vi "TIMER_VI.vi"(7 "simulazione":bool, 8 "error in (no error)":errorcluster, 11 "Queue Name":string) -> (0 "error out":errorcluster, 2 "Stopped":bool)   [LabVIEW 2019]
uses:
  Globals.vi
panel:
  out "# elements in queue":i32
  out "Elapsed Time (s)":dbl
  out "STATO":string
  out "LOOP TIME (ms)":u32
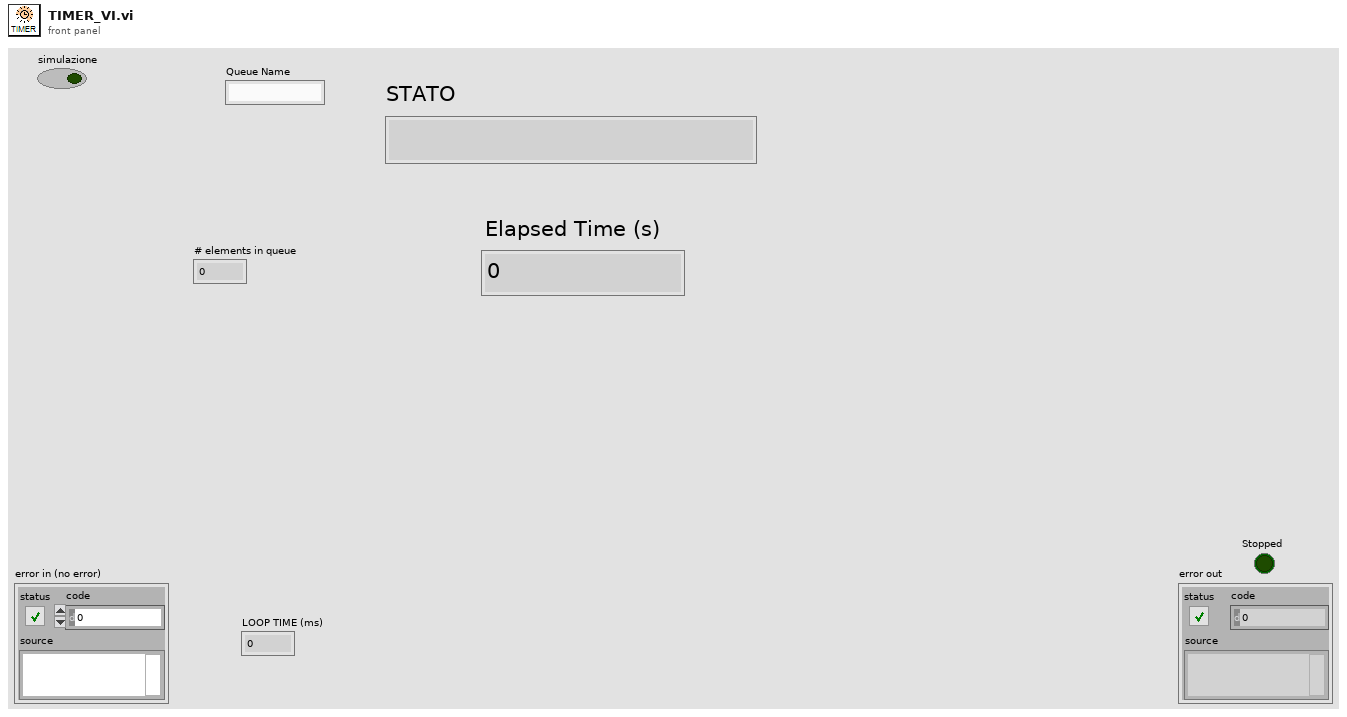
[diagram p1: front panel]
types:
  T1 = cluster{"Array of elements":cluster{"String":string, "variant":variant}[], "Single element":cluster{"String":string, "variant":variant}, "enque at\nopposite end (F)":bool, "no replications (F)":bool}
  T2 = enum32{"Invalid", "Standard", "Closed", "Hidden", "Minimized", "Maximized"}
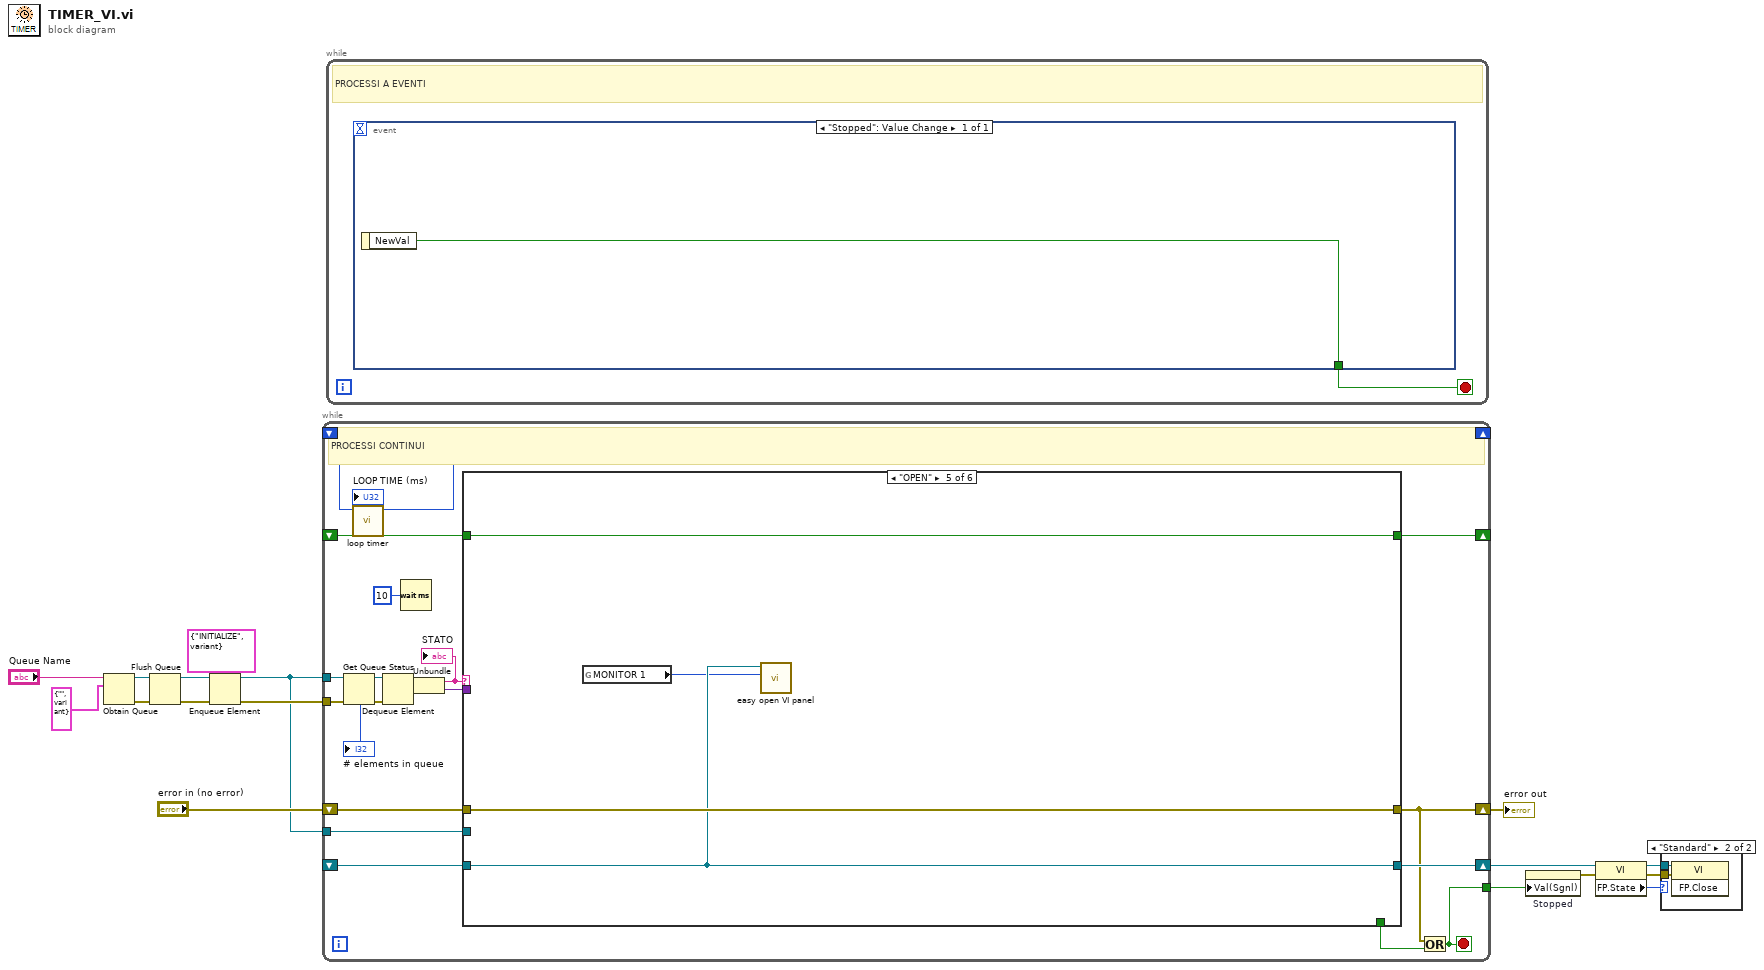
[diagram p0: block diagram]
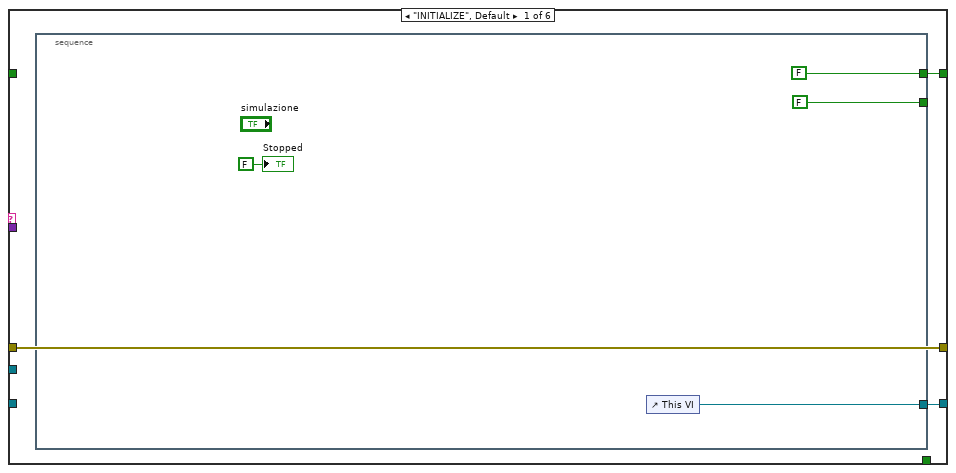
[diagram p3: hidden frame]
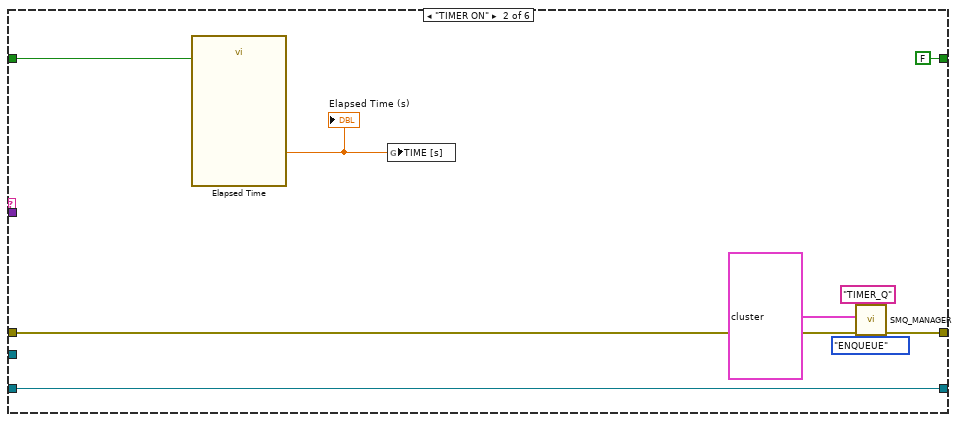
[diagram p4: hidden frame]
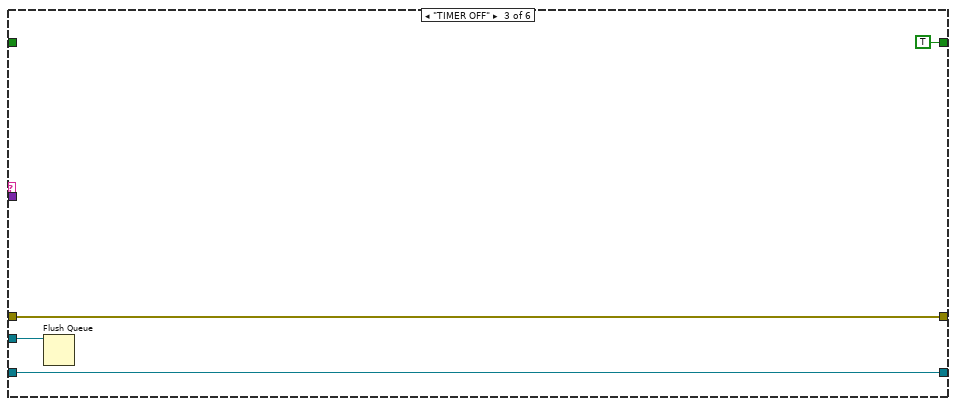
[diagram p5: hidden frame]
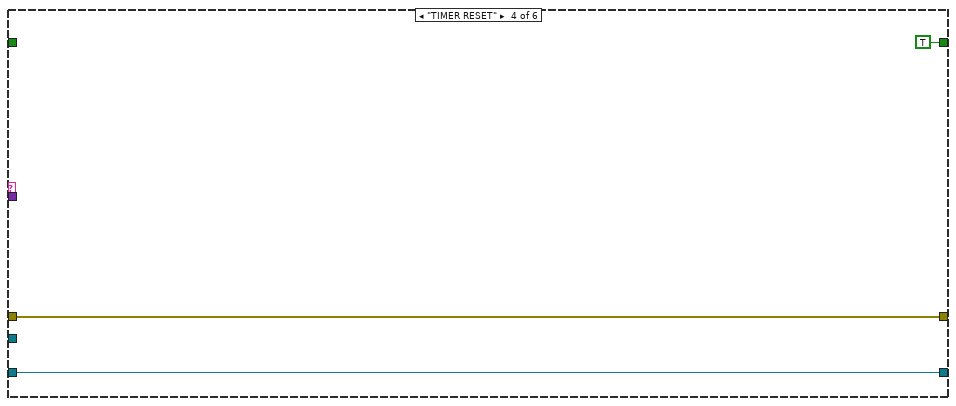
[diagram p6: hidden frame]
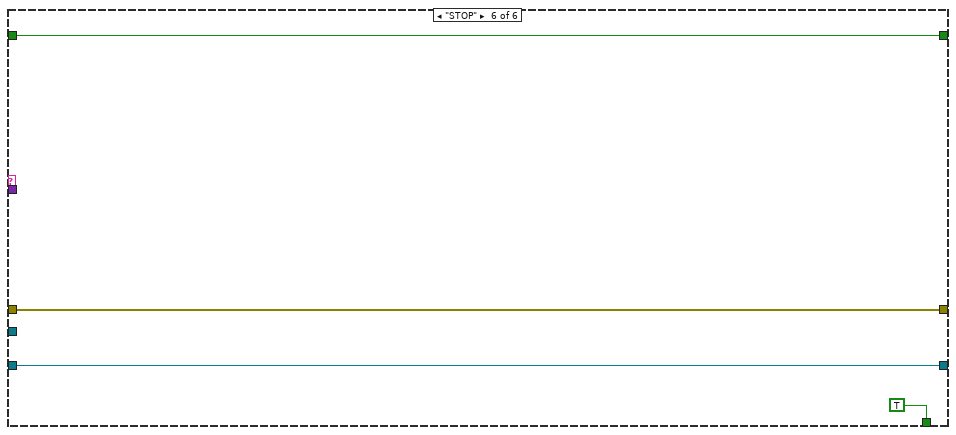
[diagram p7: hidden frame]
diagram:
  n1 = Obtain Queue(name (unnamed)="Queue Name", element data type=cluster{"String":string, "variant":variant} {"String"="", "variant"=variant} ("element")) -> (queue out=w6:refnum<queue>, error out=w5:errorcluster)  [unwired: 3 in, 1 out]
  n2 = Flush Queue(queue=w6, error in (no error)=w5) -> (queue out=w3:refnum<queue>, error out=w2:errorcluster)  [unwired: 1 out]
  n3 = Enqueue Element(queue=w3, element=cluster{"String":string, "variant":variant} {"String"="INITIALIZE", "variant"=variant}, error in (no error)=w2) -> (queue out=w1:refnum<queue>, error out=w7:errorcluster)  [unwired: 1 in, 1 out]
  n4 = while {
    shift-right: [w38] -> _
    shift-left: _ -> [w37]
    shift-right: [w35] -> w10
    shift-left: _ -> [w34]
    shift-right: [w31] -> w13
    shift-left: "error in (no error)" -> [w33]
    tunnel: w1 -> [w23]
    tunnel: w7 -> [w22]
    tunnel: [w28] -> w14
    shift-right: [w26] -> _
    shift-left: _ -> [w25]
    tunnel: w1 -> [w24]
    stop <- w28 stop-if-true
    # "PROCESSI CONTINUI"
    n5 = Get Queue Status(queue=w23, error in (no error)=w22) -> (queue out=w20:refnum<queue>, error out=w21:errorcluster, # elements in queue=→"# elements in queue":i32)  [unwired: 1 in, 5 out]
    n6 = call <userlib>:"loop timer.vi"("millisecond timer IN"=w37) -> ("millisecond timer OUT"=w38:u32, "LOOP TIME (ms)"=→"LOOP TIME (ms)":u32)  [unwired: 9 in]
    n7 = Dequeue Element(queue=w20, error in (no error)=w21) -> (element=w30:cluster{"String":string, "variant":variant})  [unwired: 1 in, 3 out]
    n8 = Wait (ms)(milliseconds to wait=u32 10) -> ()  [unwired: 1 out]
    n9 = Unbundle(w30) -> ("String"=w27:string, "variant"=w29:variant)
    "STATO" <- w27
    n10 = case shown="\"OPEN\"" w27 {
      tunnel: [_ _ _ _ _ TRUE] -> w32
      tunnel: [w41 w54 w58 w61 w64 w68] -> w35
      tunnel: w34 -> [_ w54 w58 w61 w64 w68]
      tunnel: w33 -> [w40 w50 w57 w60 w65 w67]
      tunnel: [w40 w51 w57 w60 w65 w67] -> w31
      tunnel: w29 -> [_ _ _ _ _ _]
      tunnel: [w39 FALSE TRUE TRUE w63 w66] -> w26
      tunnel: w25 -> [_ w48 _ _ w63 w66]
      tunnel: w24 -> [_ _ w56 _ _ _]
      frame "INITIALIZE", Default {
        n11 = stacked-sequence {
          tunnel: [w45] -> w41
          tunnel: [FALSE] -> w39
          tunnel: [FALSE] -> _
          frame #0 {
            n12 = control-ref of="This VI"() -> (w45:refnum<vi>)
            "Stopped" <- FALSE ("Stop")
          }
        }
      }
      frame "TIMER ON" {
        n13 = call "Elapsed Time"("Reset"=w48) -> ("Elapsed Time (s)"=w46:dbl)  [unwired: 11 in, 7 out]
        "Elapsed Time (s)" <- w46
        n14 = global write "Globals.vi" "TIME [s]"(w46) -> ()
        n15 = call <userlib>:"SMQ_MANAGER.vi"("Function"=enum16{"INITIALIZE", "ENQUEUE", "STOP ALL"}."ENQUEUE", "Queue name"="TIMER_Q", "error in (no error)"=w50, "Enqueue cluster"=T1 {"Array of elements"=[], "Single element"={"String"="TIMER ON", "variant"=variant}, "enque at\nopposite end (F)"=FALSE, "no replications (F)"=FALSE}) -> ("error out"=w51:errorcluster)  [unwired: 7 in]
      }
      frame "TIMER OFF" {
        n16 = Flush Queue(queue=w56) -> ()  [unwired: 1 in, 3 out]
      }
      frame "TIMER RESET" {
      }
      frame "OPEN" {
        n17 = global read "Globals.vi" "MONITOR 1"() -> (w62:u8)
        n18 = call <userlib>:"easy open VI panel.vi"("Monitor(1)"=w62, "VI in"=w64) -> ()  [unwired: 9 in, 1 out]
      }
      frame "STOP" {
      }
    }
    n19 = Or(x=w31, y=w32) -> (x .or. y?=w28:bool)
  }
  "error out" <- w13
  n20 = while {
    stop <- w70 stop-if-true
    # "PROCESSI A EVENTI"
    n21 = event shown="[0] \"Stopped\": Value Change" {
      selector: _ -> [_]
      dyn-events: _ -> [_]
      timeout: _ -> [_]
      tunnel: [w71] -> w70
      event "Stopped": Value Change {
        n22 = event-data() -> ("NewVal"=w71:bool)  [unwired: 1 in]
      }
    }
  }
  n23 = property on="Stopped" class="Bool (strict)"("Val(Sgnl)"=w14) -> (error out=w9:errorcluster)  [unwired: 2 in, 1 out]
  n24 = property class="VI"(reference=w10, error in=w9) -> (reference out=w12:refnum<vi>, error out=w8:errorcluster, "FP.State"=w11:T2)
  n25 = case shown="\"Standard\"" w11 {
    tunnel: w12 -> [_ w73]
    tunnel: w8 -> [_ w72]
    frame "Invalid", Default {
    }
    frame "Standard" {
      n26 = invoke class="VI" method="FP.Close"(reference=w73, error in=w72) -> ()  [unwired: 1 in, 3 out]
    }
  }
